vi "Init_child_VI.vi"(8 "error in (no error)":errorcluster, 10 "Ref VI":refnum<vi>, 11 "Control-Client in":refnum<class "Control-Client.lvclass">) -> (0 "error out":errorcluster, 3 "Control-Client out":refnum<class "Control-Client.lvclass">)   [LabVIEW 2019, in "Control-Client.lvclass"]
uses:
  Control-Client.lvclass
  Control-Client.lvclass/Control-Client.ctl
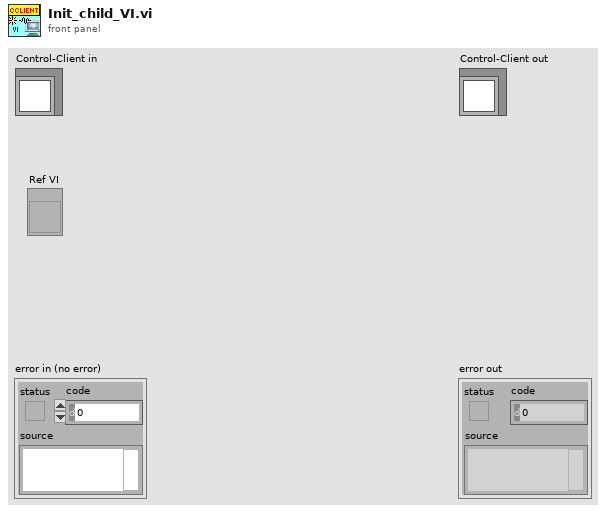
[diagram p1: front panel]
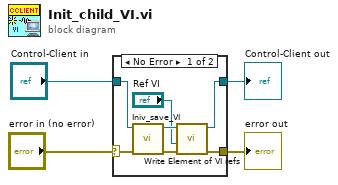
[diagram p0: block diagram]
diagram:
  n1 = case shown="No Error" "error in (no error)" {
    selector: "error in (no error)" -> [w10 w13]
    tunnel: [w5 w13] -> w3
    tunnel: [w8 w12] -> w1
    tunnel: "Control-Client in" -> [w11 w12]
    frame No Error {
      n2 = call "Iniv_save_VI.vi"("error in (no error)"=w10, "Control-Client in"=w11) -> ("error out"=w6:errorcluster, "Control-Client out"=w9:refnum<class "Control-Client.lvclass">)  [unwired: 8 in]
      n3 = call "Write Element of VI refs.vi"("error in (no error)"=w6, "vi reference"="Ref VI", "Control-Client in"=w9) -> ("error out"=w5:errorcluster, "Control-Client out"=w8:refnum<class "Control-Client.lvclass">)  [unwired: 7 in]
    }
    frame Error {
    }
  }
  "error out" <- w3
  "Control-Client out" <- w1
